vi "UI_Set_Slider_values_when_online.vi"(8 "error in (no error)":errorcluster, 9 "Online? (F)":bool, 10 "Since track start":dbl, 11 "All references":T1) -> (0 "error out":errorcluster)   [LabVIEW 2018, in "Tracker.lvlib"]
uses:
  Tracker.lvlib
  Controls/CTL_All_References.ctl
  Common/Typedefs/CTL_Controls_References.ctl
  Common/Typedefs/CTL_Indicators_References.ctl
  Common/Typedefs/CTL_Panes_and_VIs_References.ctl
  Common_Resources.lvlib
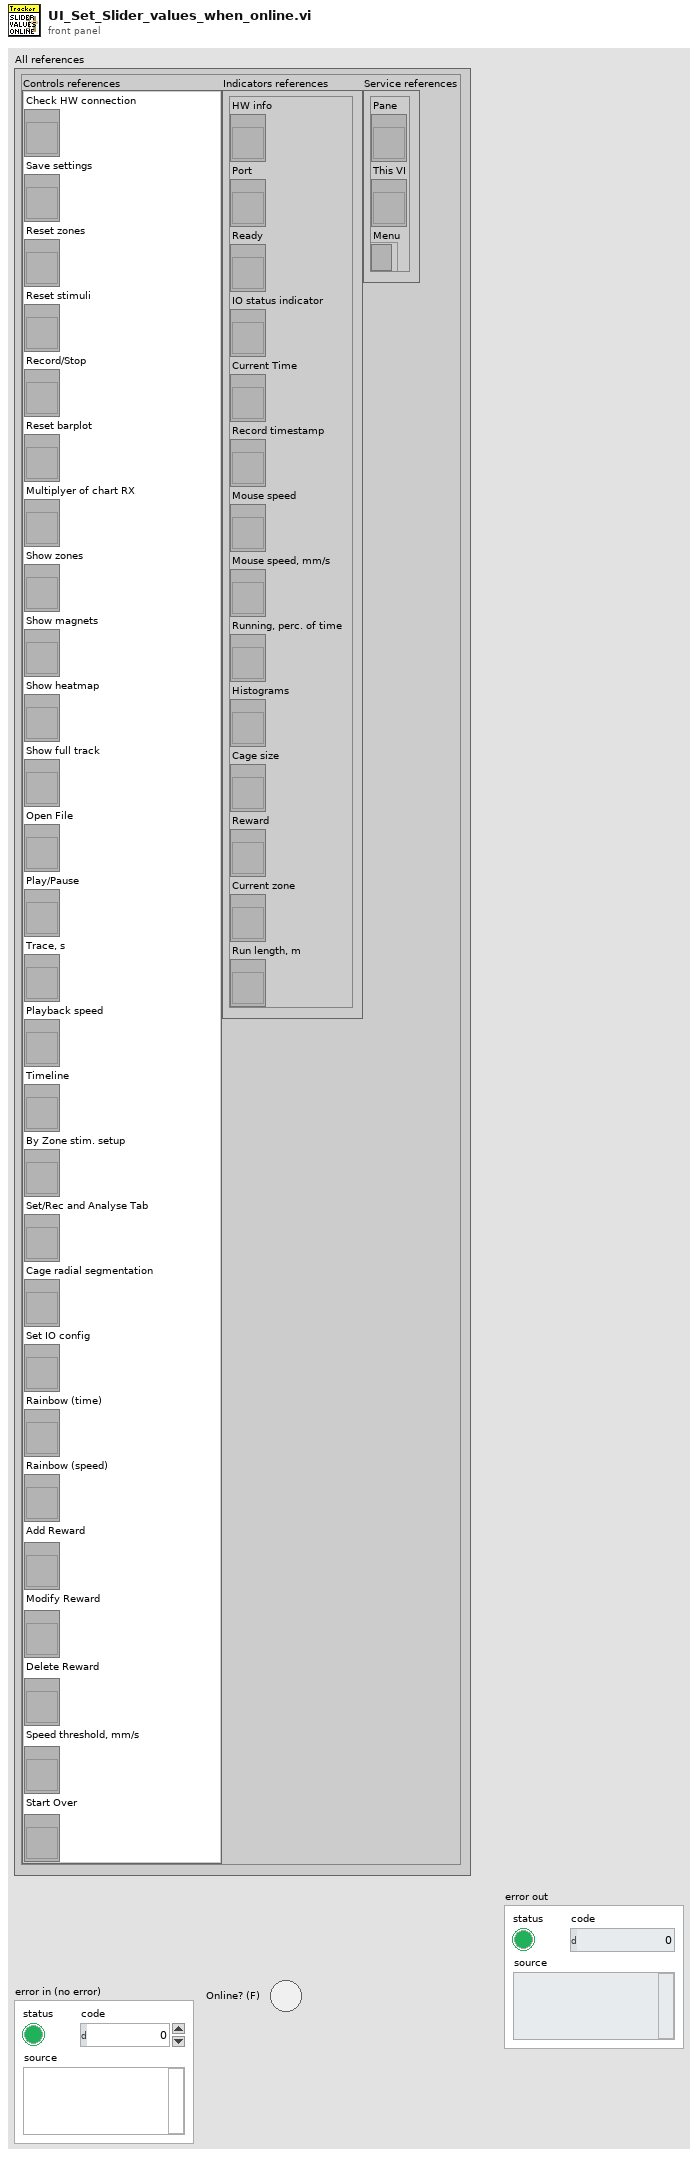
[diagram p1: front panel]
types:
  T1 = typedef "Common_Resources.lvlib/CTL_All_References.ctl" = cluster{"Controls references":T2, "Indicators references":T3, "Service references":T4}
  T2 = typedef "Common_Resources.lvlib/CTL_Controls_References.ctl" = cluster{"Check HW connection":refnum<vi>, "Save settings":refnum<vi>, "Reset zones":refnum<vi>, "Reset stimuli":refnum<vi>, "Record/Stop":refnum<vi>, "Reset barplot":refnum<vi>, "Multiplyer of chart RX":refnum<vi>, "Show zones":refnum<vi>, "Show magnets":refnum<vi>, "Show heatmap":refnum<vi>, "Show full track":refnum<vi>, "Open File":refnum<vi>, "Play/Pause":refnum<vi>, "Trace, s":refnum<vi>, "Playback speed":refnum<vi>, "Timeline":refnum<vi>, "By Zone stim. setup":refnum<vi>, "Set/Rec and Analyse Tab":refnum<vi>, "Cage radial segmentation":refnum<vi>, "Set IO config":refnum<vi>, "Rainbow (time)":refnum<vi>, "Rainbow (speed)":refnum<vi>, "Add Reward":refnum<vi>, "Modify Reward":refnum<vi>, "Delete Reward":refnum<vi>, "Speed threshold, mm/s":refnum<vi>, "Start Over":refnum<vi>}
  T3 = typedef "Common_Resources.lvlib/CTL_Indicators_References.ctl" = cluster{"HW info":refnum<vi>, "Port":refnum<vi>, "Ready":refnum<vi>, "IO status indicator":refnum<vi>, "Current Time":refnum<vi>, "Record timestamp":refnum<vi>, "Mouse speed":refnum<vi>, "Mouse speed, mm/s":refnum<vi>, "Running, perc. of time":refnum<vi>, "Histograms":refnum<vi>, "Cage size":refnum<vi>, "Reward":refnum<vi>, "Current zone":refnum<vi>, "Run length, m":refnum<vi>}
  T4 = typedef "Common_Resources.lvlib/CTL_Panes_and_VIs_References.ctl" = cluster{"Pane":refnum<vi>, "This VI":refnum<vi>, "Menu":refnum<k9>}
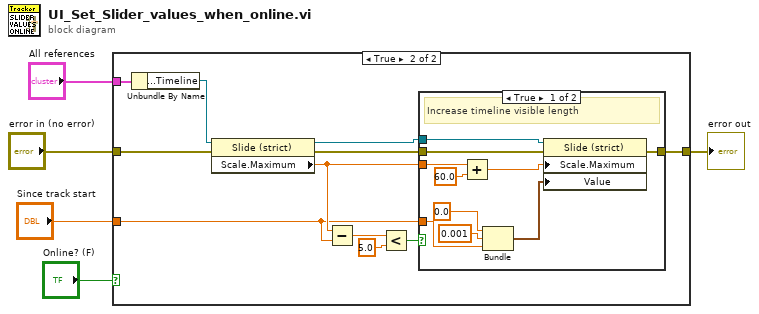
[diagram p0: block diagram]
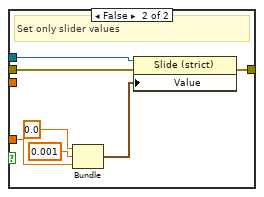
[diagram p3: hidden frame]
diagram:
  n1 = case shown="True" "Online? (F)" {
    tunnel: [w6 w16] -> w5
    tunnel: "Since track start" -> [_ w7]
    tunnel: "error in (no error)" -> [w6 w10]
    tunnel: "All references" -> [_ w8]
    frame False {
    }
    frame True {
      n2 = Unbundle By Name(w8) -> ("Controls references.Timeline"=w9:refnum<vi>)
      n3 = property class="Slide (strict)"(reference=w9, error in=w10) -> (reference out=w17:refnum<vi>, error out=w15:errorcluster, "Scale.Maximum"=w14:dbl)
      n4 = Subtract(x=w14, y=w7) -> (x-y=w11:dbl)
      n5 = Less?(x=w11, y=5.0) -> (x < y?=w13:bool)
      n6 = case shown="True" w13 {
        tunnel: w14 -> [w27 _]
        tunnel: w15 -> [w25 w34]
        tunnel: [w23 w33] -> w16
        tunnel: w17 -> [w22 w32]
        tunnel: w7 -> [w19 w29]
        frame True {
          # "Increase timeline visible length"
          n7 = Add(x=w27, y=60.0) -> (x+y=w24:dbl)
          n8 = Bundle(0.0, 0.001, "Since track start"=w19) -> (w18:cluster{dbl, dbl, "Since track start":dbl})  [unwired: 1 in]
          n9 = property class="Slide (strict)"(reference=w22, error in=w25, "Scale.Maximum"=w24, "Value"=w18) -> (error out=w23:errorcluster)  [unwired: 1 out]
        }
        frame False {
          # "Set only slider values"
          n10 = Bundle(0.0, 0.001, "Since track start"=w29) -> (w28:cluster{dbl, dbl, "Since track start":dbl})  [unwired: 1 in]
          n11 = property class="Slide (strict)"(reference=w32, error in=w34, "Value"=w28) -> (error out=w33:errorcluster)  [unwired: 1 out]
        }
      }
    }
  }
  "error out" <- w5
